vi "Launch Root Digital Reader Actor.vi"(8 "error in (no error)":errorcluster, 10 "Digital Reader Actor":refnum<class "Digital Reader.lvclass">) -> (0 "error out":errorcluster, 1 "Digital Input Current Values":refnum<queue>, 2 "Actor's Enqueuer":refnum<class "Message Enqueuer.lvclass">)   [LabVIEW 2024, in "DAQmx Actor.lvlib" / "Digital Reader.lvclass"]
uses:
  Digital Reader.lvclass
  Digital Reader.lvclass/Digital Reader.ctl
  <vilib>/ActorFramework/Actor/Actor.lvclass
  C:/Users/uspoaotto/OneDrive - Oregon Tool/Desktop/working copies/DAQmxActor/src/DAQmx Actor/DAQmx Actor/DAQmx Actor.lvclass
  C:/Program Files (x86)/National Instruments/LabVIEW 2024/vi.lib/ActorFramework/Actor/Actor.lvclass
  C:/Users/uspoaotto/OneDrive - Oregon Tool/Desktop/working copies/DAQmxActor/src/DAQmx Actor/Digital Reader/Digital Reader.lvclass
  <vilib>/ActorFramework/Message Enqueuer/Message Enqueuer.lvclass
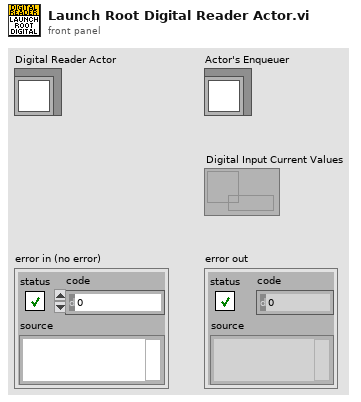
[diagram p1: front panel]
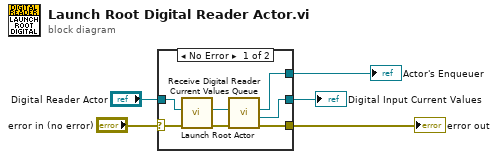
[diagram p0: block diagram]
diagram:
  n1 = case shown="No Error" "error in (no error)" {
    selector: "error in (no error)" -> [w6 w13]
    tunnel: "Digital Reader Actor" -> [w12 _]
    tunnel: [w10 w13] -> w4
    tunnel: [w8 _] -> w3
    tunnel: [w7 _] -> w2
    frame No Error {
      n2 = call <vilib>:"Launch Root Actor.vi"("error in (no error)"=w6, "Actor"=w12) -> ("error out"=w11:errorcluster, "Actor's Enqueuer"=w9:refnum<class "Message Enqueuer.lvclass">)  [unwired: 8 in]
      n3 = call "Receive Digital Reader Current Values Queue.vi"("error in (no error)"=w11, "Message Enqueuer"=w9) -> ("error out"=w10:errorcluster, "Digital Input Current Values"=w7:refnum<queue>, "Message Enqueuer out"=w8:refnum<class "Message Enqueuer.lvclass">)  [unwired: 7 in]
    }
    frame Error {
    }
  }
  "error out" <- w4
  "Actor's Enqueuer" <- w3
  "Digital Input Current Values" <- w2
